vi "收集数据ICRA2024测试椭圆分裂加PID控制.vi"() -> ()   [LabVIEW 2018]
doc: "Demonstrates the use of the Network Streams functions to send LED status to the myRIO target."
uses:
  <vilib>/ErrorRing/Error Ring.xnode
  <vilib>/vision/NI_Vision_Development_Module.lvlib
panel:
  in  "布尔":bool
  in  "ribbon磁场开关":bool=TRUE
  out "控制量":dbl
  in  "期望ratio":dbl=5.0
  in  "拉伸的增益":dbl=10.0
  in  "收缩的增益":dbl=5.0
  in  "predefined control":dbl=5.0
  out "面积":sgl[](array[numeric])
  out "面积":sgl
  out "数据总":dbl[][](array[numeric])
  out "i":i32[](array[numeric])
  out "aspect ratio":dbl[](array[numeric])
  out "D2":i32[](array[numeric])
  out "D1":i32[](array[numeric])
  out "field ratio":sgl[](array[numeric])
  out "field ratio":sgl=4.0
  out "时间":i32
  in  "打开数据记录":bool
  out "aspect ratio":dbl
  out "D2":i32
  out "D1":i32
  out "二值图":T1(plugin-control)
  in  "Search Rect (entire image)":T2={"Left"=200, "Top"=120, "Right"=2000, "Bottom"=1920, "Rotation"=0.0} {"Rotation" format="%.2f"; "Left" scale=0.0..1024.0; "Right" scale=0.0..1024.0}
  out "备用的椭圆角度":sgl
  in  "Number of Erosion":i32=10
  out "Image 7":T1(plugin-control)
  in  "Acquisition Control::Acquisition Frame Rate":dbl=19.50304412841797 min=1.4211589097976685 max=44.94382095336914
  out "Stopped":bool
  in  "Stop (F) 2":bool caption="Stop (F)"
  out "Objects 2":T3(array[cluster]) {"Aspect Ratio" format="%.2f"; "Orientation" format="%.2f"; "Area" format="%.2f"; "Object Center"."Y" format="%.2f"; "Object Center"."X" format="%.2f"}
  in  "Settings 2":T4={"Objects"=0, "Threshold"=128, "Reject Border"=FALSE, "Fill Holes"=FALSE, "Min Object Size"=FALSE, "Min Size"=20000, "Max Object Size"=FALSE, "Max Size"=100, "Show Search Area"=FALSE, "Show Center"=TRUE, "Show Bounding Box"=TRUE} {"Objects" items=["Bright Objects", "Dark Objects"]; "Threshold" min=1 max=999999999 step=1; "Max Size" min=1 max=999999999 step=1; "Min Size" min=1 max=999999999 step=1}
  in  "Range 2":cluster{"Lower value":sgl, "Upper value":sgl}={"Lower value"=0.0, "Upper value"=230.0} {"Upper value" format="%.2f"; "Lower value" format="%.2f"}
  in  "Pause":bool
  out "Array":dbl[](array[numeric])
  in  "Parameter Settings":T5(tab)=enum."Ribbon Oscillating Field" caption="Field Types"
  in  "fg":dbl
  in  "pg":dbl
  in  "dg":dbl
  in  "Ag":dbl
  in  "AoOF":dbl
  in  "fo":sgl
  in  "do":sgl
  in  "oo":sgl
  in  "po":sgl
  in  "cc":sgl
  in  "pc":sgl
  in  "wc":sgl
  in  "dc":sgl
  in  "Ac":dbl
  in  "pr":sgl
  in  "Ar":dbl=8.0
  in  "wr":sgl=18.0
  in  "dr":sgl
  in  "Dis phase step":dbl
  in  "Dis phase frequency (Hz)":dbl
  in  "Dis tumbling frequency (Hz)":dbl
  in  "Dis strength(mT)":dbl
  in  "Swa strength (mT)":dbl
  in  "Swa frequency (Hz)":dbl
  in  "Swa pitch angle (deg)":dbl
  in  "Swa direction angle (deg)":dbl
  in  "Swa ratio":dbl=1.0
  in  "Pitch Angle (rotating around Constant, deg)":dbl
  in  "Ratio (A/C)":sgl=4.0
  in  "Direction Angle (deg)":sgl
  in  "Pitch Angle (rotating around Origin, deg)":sgl
  in  "Frequency (Hz)":sgl=10.0
  in  "Strength (mT)":dbl=10.0
  in  "Ar 2":dbl=5.0 caption="Ar"
  in  "ratio":sgl=1.0
  in  "运动方向":sgl
  in  "长轴方向":sgl
  in  "wr  2":sgl=8.0
  in  "速度大小":sgl
  out "Numeric 5":i32
  in  "Stop":bool
  out "error out":errorcluster
  in  "Target IP Address":string="172.22.11.2"
  # "Overview: Magnetic field calculation, and send parameters to myRIO\nInstructions:\n1. Verify the value of Target IP Address. Set Visa resource name.\n2. Ensure RT Main.vi is already running. \n3. Run this VI. Set parameters of magnetic field."
  # "Strength (mT)"
  # "Pitch Angle (deg)"
  # "Direction Angle (deg)"
  # "Frequency (Hz)"
  # "Strength (mT)"
  # "Oscilation Frequency (Hz)"
  # "Oscilation Angle (deg)"
  # "Pitch Angle (deg)"
  # "Direction Angle (deg)"
  # "Strength (mT)"
  # "Frequency (Hz)"
  # "Pitch Angle (deg)"
  # "Direction Angle (deg)"
  # "Conical Angle (deg)"
  # "Strength (mT)"
  # "Frequency (Hz)"
  # "Pitch Angle (deg)"
  # "Direction Angle (deg)"
  # "Strength (mT)"
  # "Tumbling Frequency (Hz)"
  # "Phase Frequency (Hz)"
  # "Phase Step"
  # "Strength (mT)"
  # "Frequency (Hz)"
  # "Pitch Angle (deg)"
  # "Direction Angle (deg)"
  # "Ratio"
  # "Strength (mT)"
  # "Frequency (Hz)"
  # "Ratio (A/C)"
  # "Direction Angle (deg)"
  # "Pitch Angle (rotating around Origin, deg)"
  # "Pitch Angle (rotating around Constant, deg)"
  # "Strength (mT)"
  # "Frequency (Hz)"
  # "Pitch Angle  (deg)"
  # "longaxis"
  # "Direction Angle (deg)"
  # "ratio (l/s)"
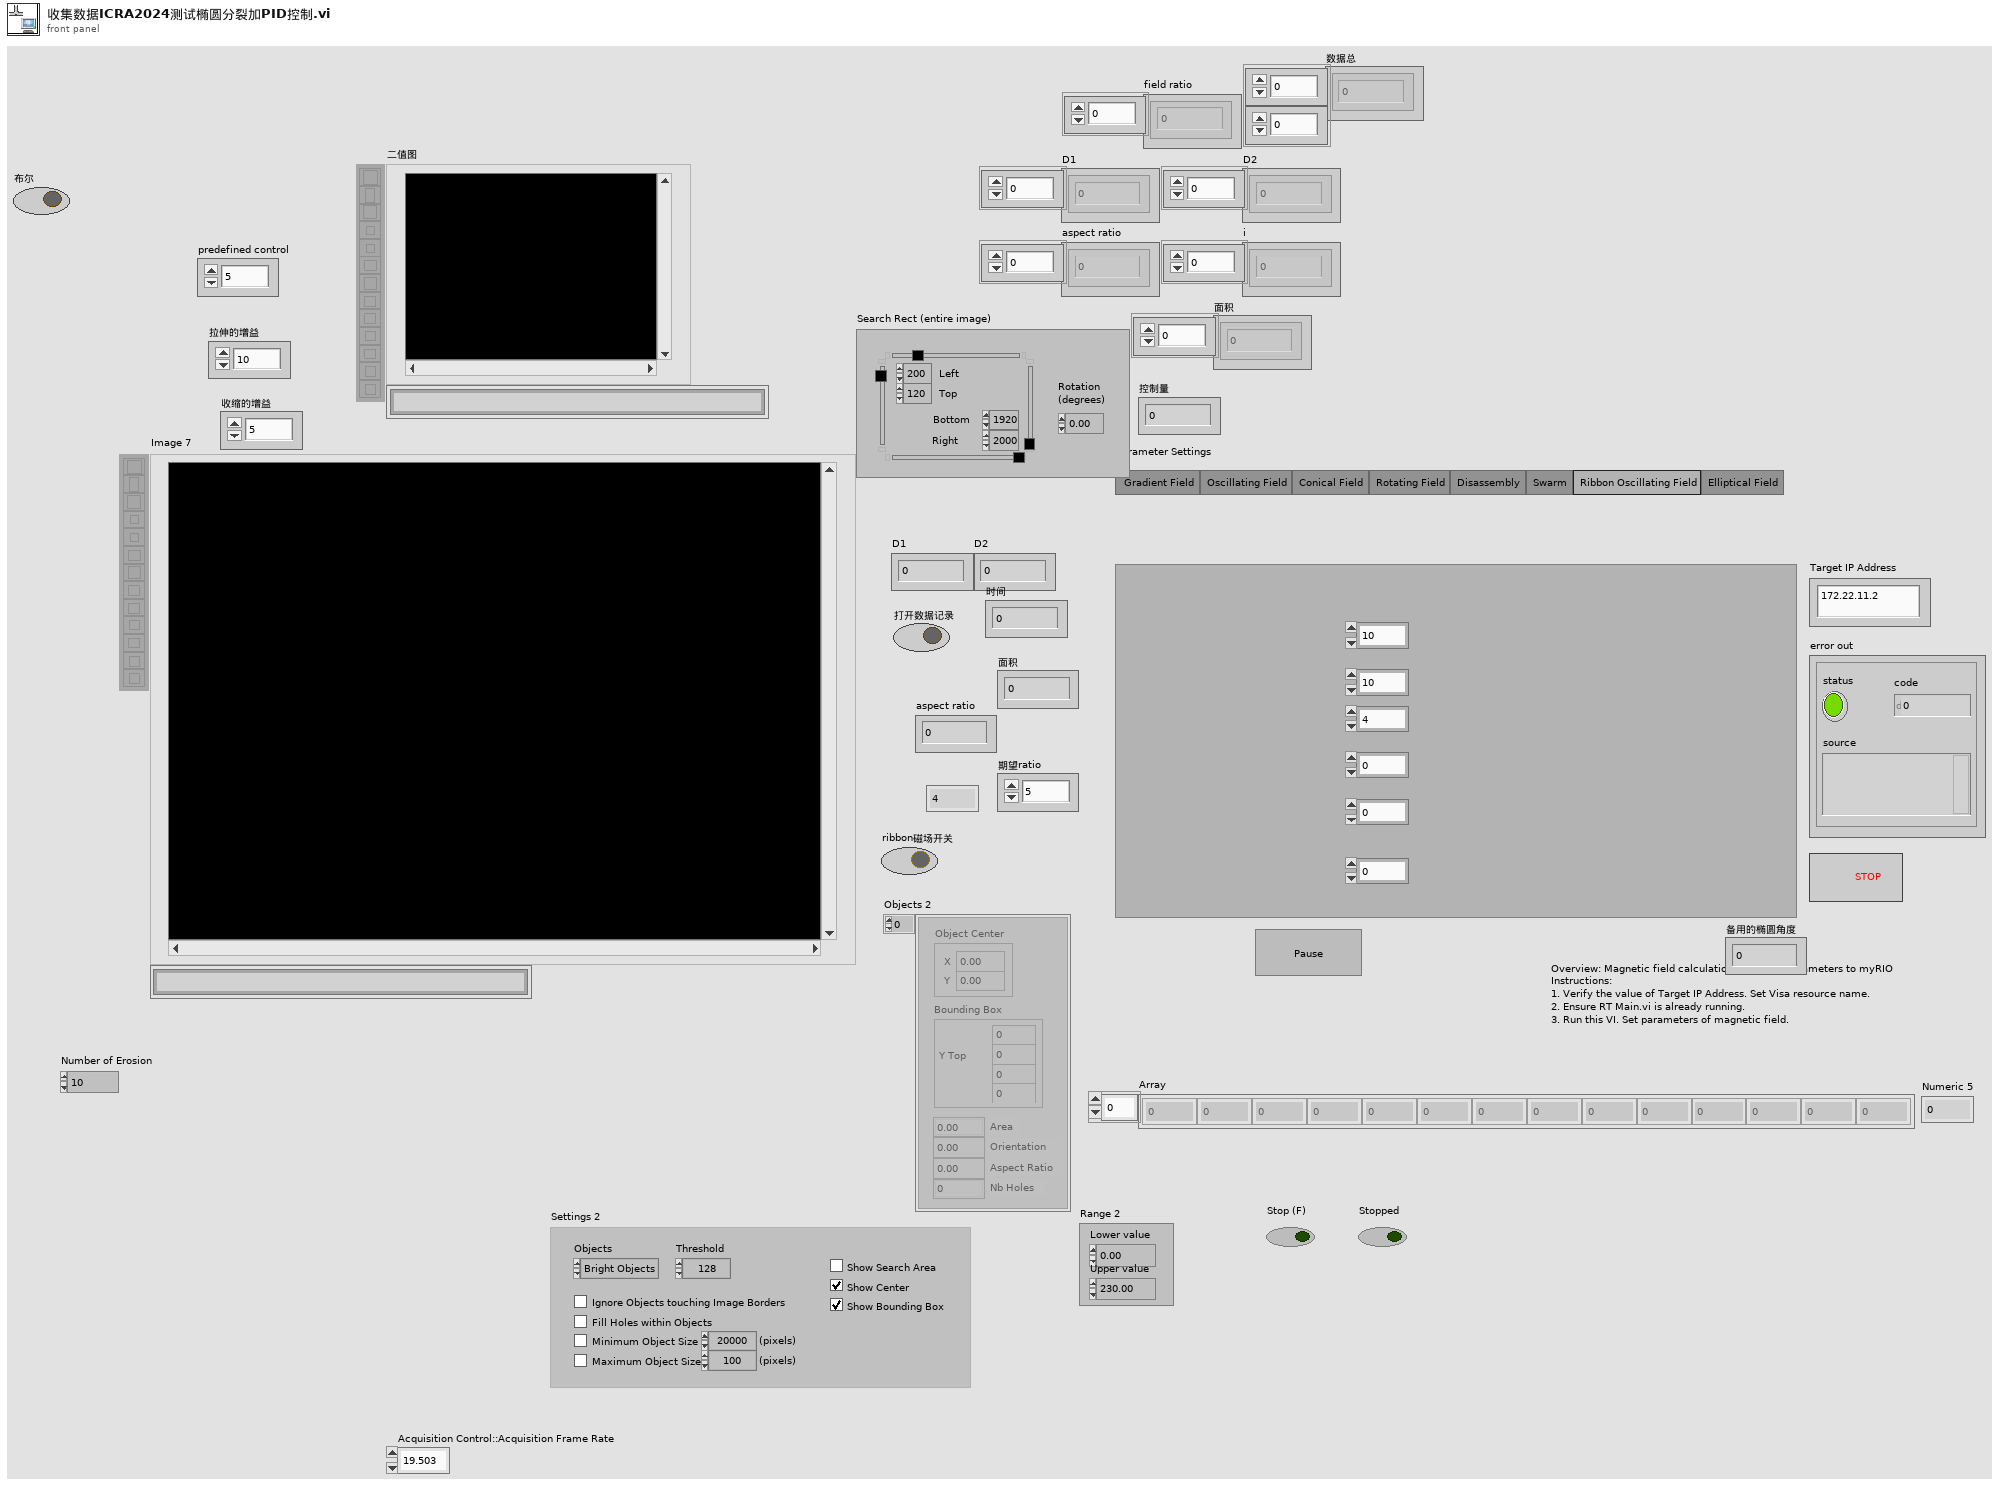
[diagram p1: front panel]
types:
  T1 = typedef "IMAQ Image.ctl" = refnum<image>
  T2 = typedef "IMAQ Rectangle" = cluster{"Left":i32, "Top":i32, "Right":i32, "Bottom":i32, "Rotation":dbl}
  T3 = cluster{"Object Center":cluster{"X":sgl, "Y":sgl}, "Bounding Box":cluster{"X Left":i32, "Y Top":i32, "X Right":i32, "Y Bottom":i32}, "Area":sgl, "Orientation":sgl, "Aspect Ratio":sgl, "Nb Holes":i32}[]
  T4 = cluster{"Objects":u16, "Threshold":i32, "Reject Border":bool, "Fill Holes":bool, "Min Object Size":bool, "Min Size":i32, "Max Object Size":bool, "Max Size":i32, "Show Search Area":bool, "Show Center":bool, "Show Bounding Box":bool}
  T5 = enum32{"Gradient Field ", "Oscillating Field", "Conical Field", "Rotating Field", "Disassembly", "Swarm", "Ribbon Oscillating Field", "Elliptical Field"}
  T6 = typedef "Image Type" = u32
  T7 = cluster{"Objects[0]":cluster{"Object Center":cluster{"X":sgl, "Y":sgl}, "Bounding Box":cluster{"X Left":i32, "Y Top":i32, "X Right":i32, "Y Bottom":i32}, "Area":sgl, "Orientation":sgl, "Aspect Ratio":sgl, "Nb Holes":i32}, "Objects[1]":cluster{"Object Center":cluster{"X":sgl, "Y":sgl}, "Bounding Box":cluster{"X Left":i32, "Y Top":i32, "X Right":i32, "Y Bottom":i32}, "Area":sgl, "Orientation":sgl, "Aspect Ratio":sgl, "Nb Holes":i32}, "Objects[2]":cluster{"Object Center":cluster{"X":sgl, "Y":sgl}, "Bounding Box":cluster{"X Left":i32, "Y Top":i32, "X Right":i32, "Y Bottom":i32}, "Area":sgl, "Orientation":sgl, "Aspect Ratio":sgl, "Nb Holes":i32}, "Objects[3]":cluster{"Object Center":cluster{"X":sgl, "Y":sgl}, "Bounding Box":cluster{"X Left":i32, "Y Top":i32, "X Right":i32, "Y Bottom":i32}, "Area":sgl, "Orientation":sgl, "Aspect Ratio":sgl, "Nb Holes":i32}, "Objects[4]":cluster{"Object Center":cluster{"X":sgl, "Y":sgl}, "Bounding Box":cluster{"X Left":i32, "Y Top":i32, "X Right":i32, "Y Bottom":i32}, "Area":sgl, "Orientation":sgl, "Aspect Ratio":sgl, "Nb Holes":i32}, "Objects[5]":cluster{"Object Center":cluster{"X":sgl, "Y":sgl}, "Bounding Box":cluster{"X Left":i32, "Y Top":i32, "X Right":i32, "Y Bottom":i32}, "Area":sgl, "Orientation":sgl, "Aspect Ratio":sgl, "Nb Holes":i32}, "Objects[6]":cluster{"Object Center":cluster{"X":sgl, "Y":sgl}, "Bounding Box":cluster{"X Left":i32, "Y Top":i32, "X Right":i32, "Y Bottom":i32}, "Area":sgl, "Orientation":sgl, "Aspect Ratio":sgl, "Nb Holes":i32}, "Objects[7]":cluster{"Object Center":cluster{"X":sgl, "Y":sgl}, "Bounding Box":cluster{"X Left":i32, "Y Top":i32, "X Right":i32, "Y Bottom":i32}, "Area":sgl, "Orientation":sgl, "Aspect Ratio":sgl, "Nb Holes":i32}, "Objects[8]":cluster{"Object Center":cluster{"X":sgl, "Y":sgl}, "Bounding Box":cluster{"X Left":i32, "Y Top":i32, "X Right":i32, "Y Bottom":i32}, "Area":sgl, "Orientation":sgl, "Aspect Ratio":sgl, "Nb Holes":i32}}
  T8 = cluster{"Object Center":cluster{"X":sgl, "Y":sgl}, "Bounding Box":cluster{"X Left":i32, "Y Top":i32, "X Right":i32, "Y Bottom":i32}, "Area":sgl, "Orientation":sgl, "Aspect Ratio":sgl, "Nb Holes":i32}
  T9 = cluster{"X Left":i32, "Y Top":i32, "X Right":i32, "Y Bottom":i32}
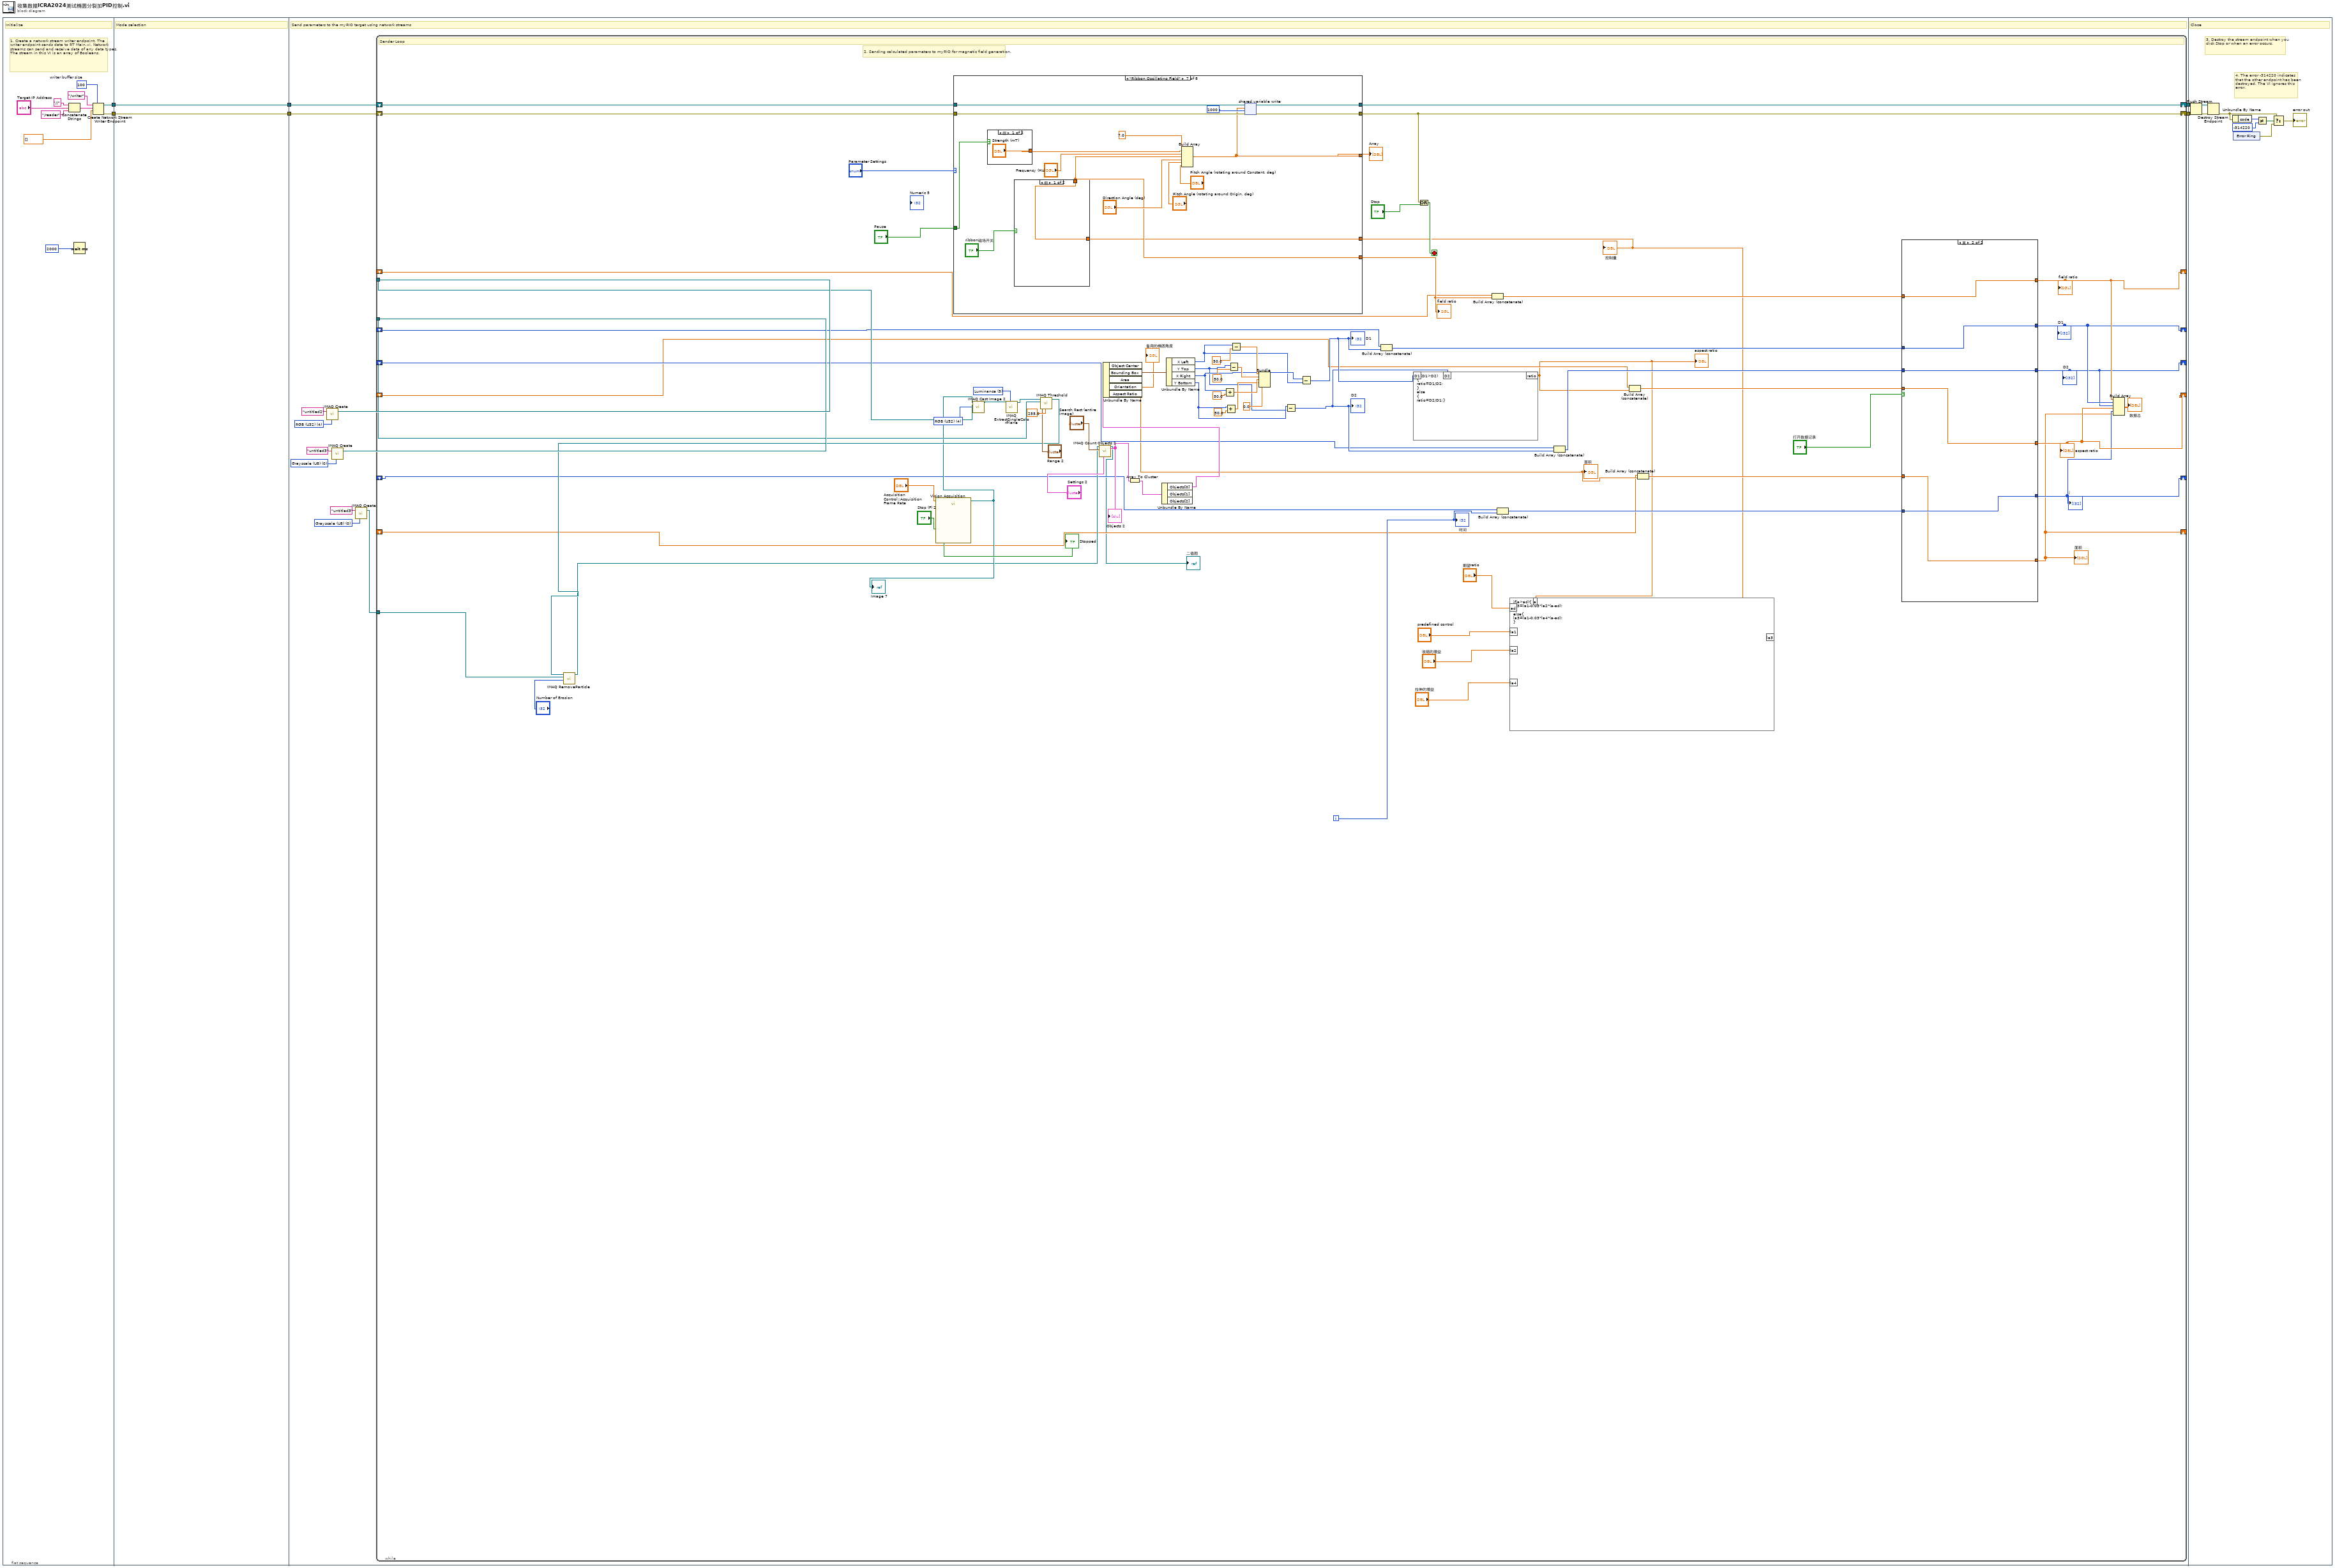
[diagram p0: block diagram]
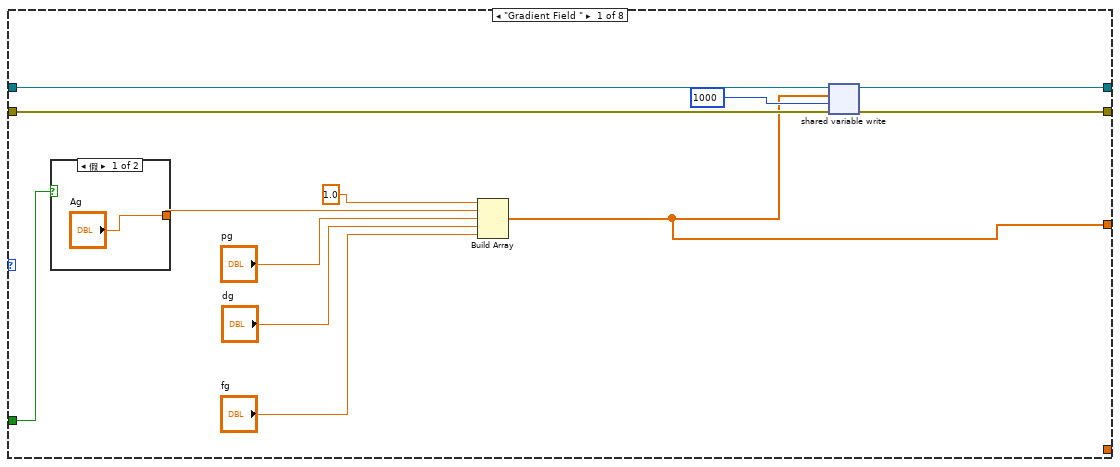
[diagram p3: hidden frame]
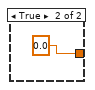
[diagram p4: hidden frame]
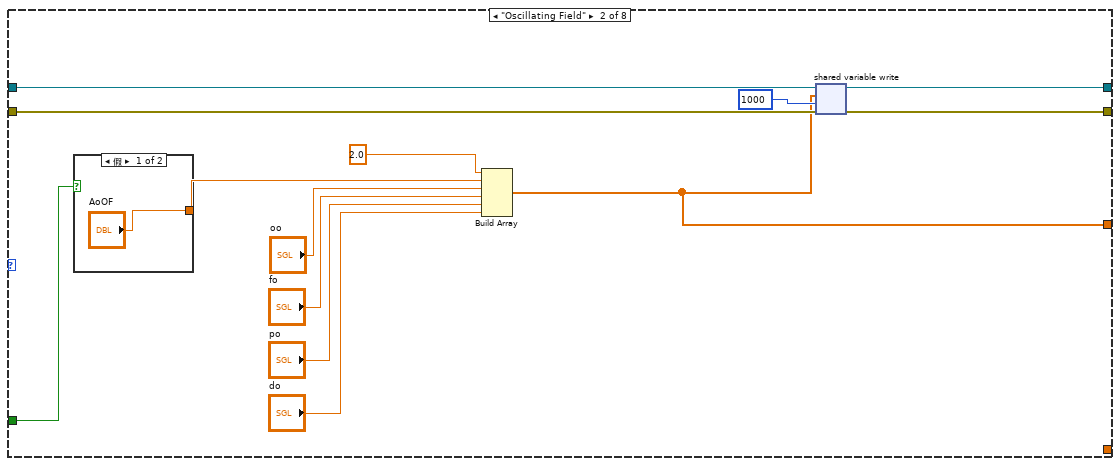
[diagram p5: hidden frame]
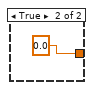
[diagram p6: hidden frame]
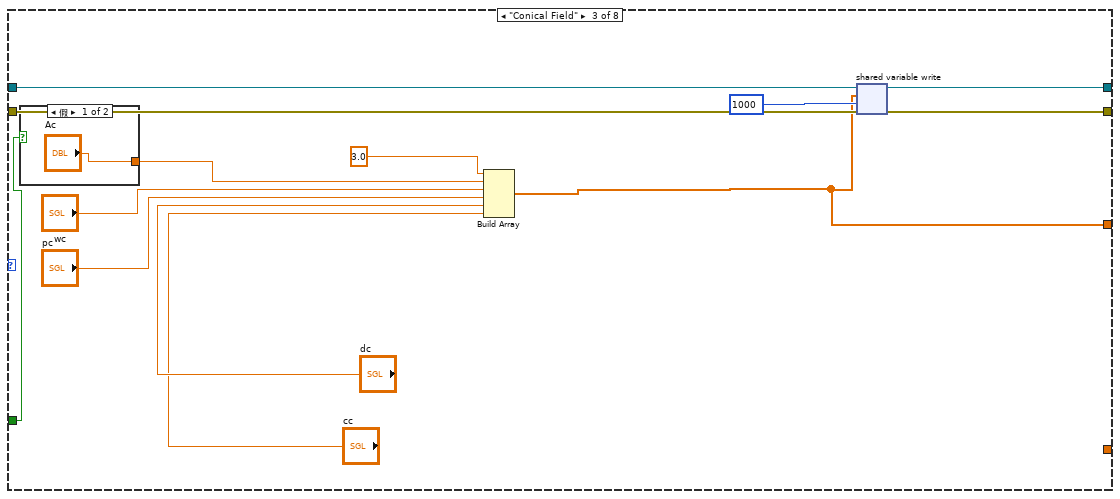
[diagram p7: hidden frame]
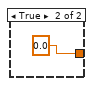
[diagram p8: hidden frame]
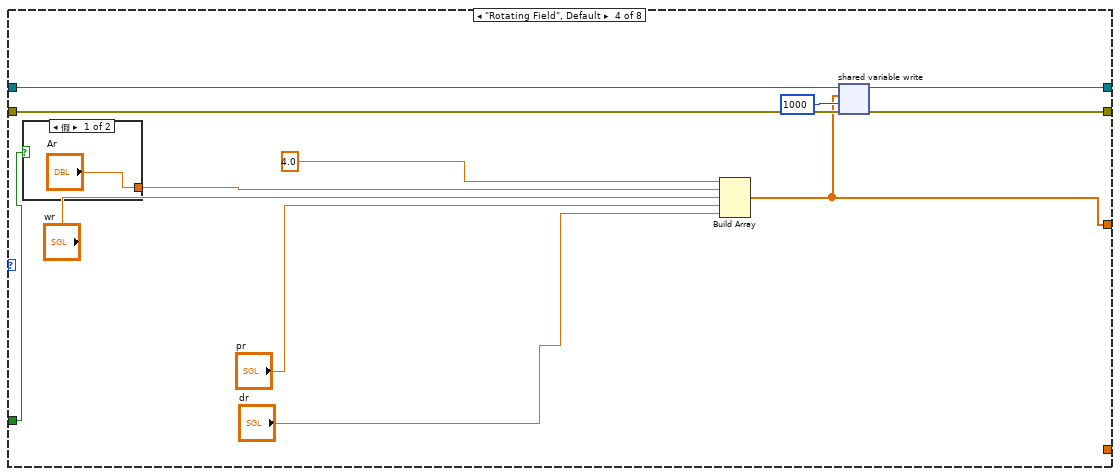
[diagram p9: hidden frame]
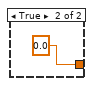
[diagram p10: hidden frame]
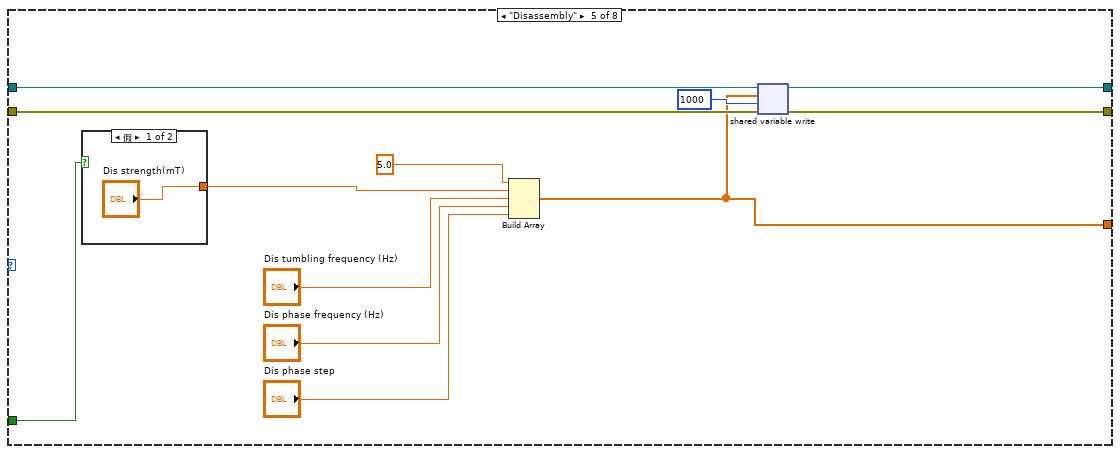
[diagram p11: hidden frame]
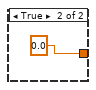
[diagram p12: hidden frame]
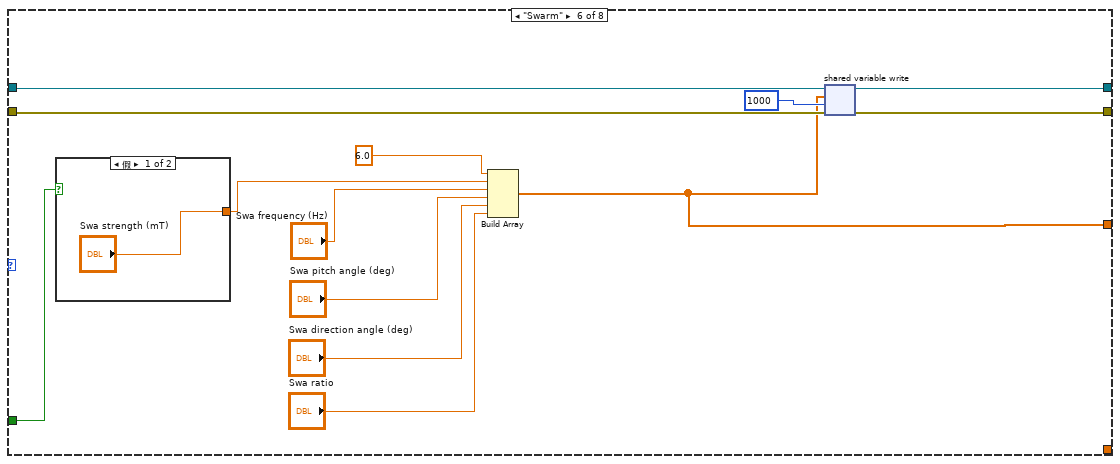
[diagram p13: hidden frame]
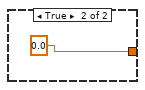
[diagram p14: hidden frame]
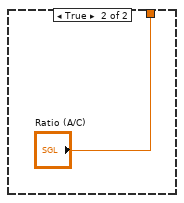
[diagram p15: hidden frame]
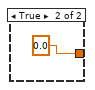
[diagram p16: hidden frame]
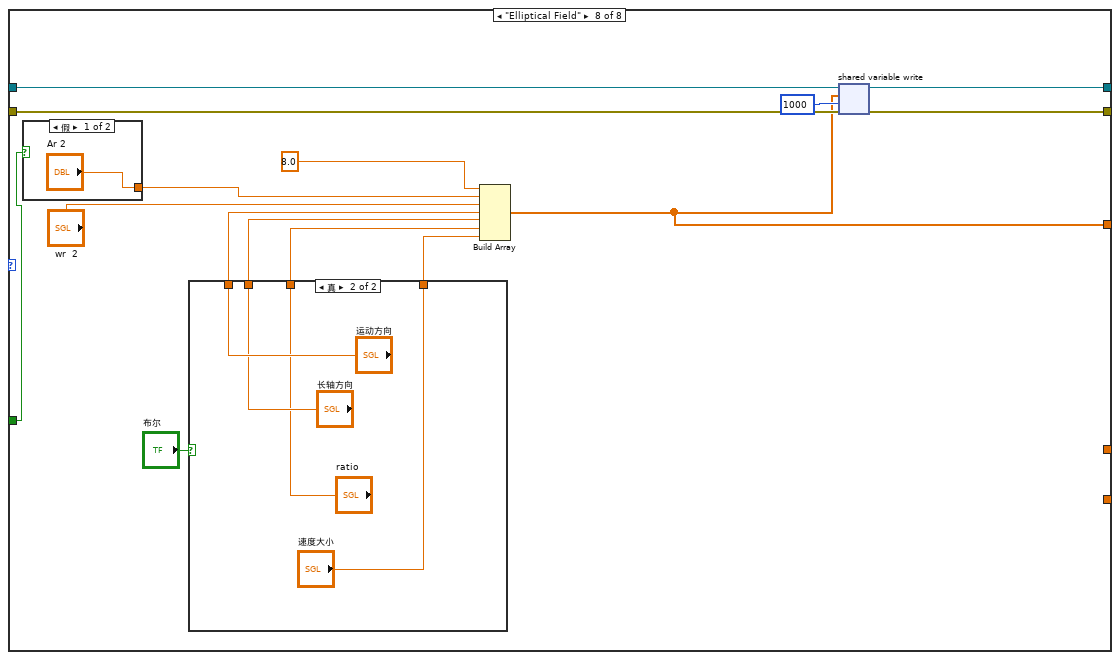
[diagram p17: hidden frame]
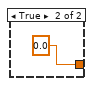
[diagram p19: hidden frame]
diagram:
  n1 = flat-sequence {
    tunnel: [w11] -> w2
    tunnel: [w10] -> w1
    tunnel: [w18] -> w4
    tunnel: [w17] -> w3
    tunnel: w1 -> [w17]
    tunnel: w2 -> [w18]
    tunnel: [w29] -> w6
    tunnel: w4 -> [w31]
    tunnel: [w28] -> w5
    tunnel: w3 -> [w30]
    tunnel: w6 -> [w252]
    tunnel: w5 -> [w249]
    frame #0 {
      w9 = 100  # writer buffer size
      # "1. Create a network stream writer endpoint. The writer endpoint sends data to RT Main.vi. Network streams can send and receive data of any data types. The stream in this VI is an array of Booleans."
      # "Initialize"
      n2 = Concatenate Strings("//", "Target IP Address", "/reader") -> (w16:string)
      n3 = Wait (ms)(milliseconds to wait=2000) -> ()  [unwired: 1 out]
      n4 = Create Network Stream Writer Endpoint(7:w9, 9:dbl[] [], 10:w16, 11:"/writer" ("reader name")) -> (0:w10:errorcluster, 3:w11:refnum<k21>)  [unwired: 3 in]
    }
    frame #1 {
      # "Mode selection"
    }
    frame #2 {
      w20 = T6 0 items=["Grayscale (U8)", "Grayscale (I16)", "Grayscale (SGL)", "Complex (CSG)", "RGB (U32)", "HSL (U32)", "RGB (U64)", "Grayscale (U16)"] ("Image Type")
      w24 = T6 0 items=["Grayscale (U8)", "Grayscale (I16)", "Grayscale (SGL)", "Complex (CSG)", "RGB (U32)", "HSL (U32)", "RGB (U64)", "Grayscale (U16)"] ("Image Type")
      w26 = T6 4 items=["Grayscale (U8)", "Grayscale (I16)", "Grayscale (SGL)", "Complex (CSG)", "RGB (U32)", "HSL (U32)", "RGB (U64)", "Grayscale (U16)"] ("Image Type")
      # "Send parameters to the myRIO target using network streams"
      n5 = call "IMAQ Create"("Image Name"="untitled2", "Image Type"=w26) -> ("New Image"=w23:T1)  [unwired: 3 in, 1 out]
      n6 = call "IMAQ Create"("Image Name"="untitled3", "Image Type"=w24) -> ("New Image"=w22:T1)  [unwired: 3 in, 1 out]
      n7 = call "IMAQ Create"("Image Name"="untitled3", "Image Type"=w20) -> ("New Image"=w19:T1)  [unwired: 3 in, 1 out]
      n8 = while {
        shift-right: [w104] -> w28
        shift-left: w30 -> [w106]
        shift-right: [w105] -> w29
        shift-left: w31 -> [w107]
        tunnel: w22 -> [w95]
        tunnel: w23 -> [w90]
        tunnel: w19 -> [w75]
        shift-right: [w48] -> _
        shift-left: _ -> [w60]
        shift-right: [w47] -> _
        shift-left: _ -> [w57]
        shift-right: [w46] -> _
        shift-left: _ -> [w54]
        shift-right: [w45] -> _
        shift-left: _ -> [w52]
        shift-right: [w44] -> _
        shift-left: _ -> [w49]
        shift-right: [w40] -> _
        shift-left: _ -> [w39]
        i -> [w51]
        stop <- w94 stop-if-true
        w89 = T6 4 items=["Grayscale (U8)", "Grayscale (I16)", "Grayscale (SGL)", "Complex (CSG)", "RGB (U32)", "HSL (U32)", "RGB (U64)", "Grayscale (U16)"] ("Image Type")
        w100 = 5 items=["Red", "Green", "Blue", "Hue", "Saturation", "Luminance", "Value", "Intensity"] ("Color Plane")
        # "2. Sending calculated parameters to myRIO for magnetic field generation."
        # "Sender Loop"
        n9 = call "Vision Acquisition"("Acquisition Control::Acquisition Frame Rate"="Acquisition Control::Acquisition Frame Rate", "Stop (F)"="Stop (F) 2") -> ("Image Out"=w67:T1, "Stopped"=→"Stopped":bool)  [unwired: 23 in, 1 out]
        "Image 7" <- w67
        n10 = call "IMAQ Cast Image 2"("Image Src"=w67, "Image Dst"=w90, "Image Type"=w89) -> ("Image Dst Out"=w91:T1)  [unwired: 11 in, 1 out]
        n11 = call "IMAQ ExtractSingleColorPlane"("Color Plane"=w100, "Image Src"=w91) -> ("Image Dst Out"=w73:T1)  [unwired: 8 in, 1 out]
        n12 = call "IMAQ Threshold"("Replace Value"=sgl 255.0, "Range"="Range 2", "Image Dst"=w95, "Image Src"=w73) -> ("Image Dst Out"=w76:T1)  [unwired: 6 in, 1 out]
        n13 = call "IMAQ RemoveParticle"("Number of Erosion"="Number of Erosion", "Image Dst"=w75, "Image Src"=w76) -> ("Image Dst Out"=w66:T1)  [unwired: 7 in, 1 out]
        n14 = call "IMAQ Count Objects 2"("Settings"="Settings 2", "Search Rect (entire image)"="Search Rect (entire image)", "Image"=w66) -> ("Image Out"=→"二值图":T1, "Objects"=w96:T3)  [unwired: 4 in, 3 out]
        "Objects 2" <- w96
        n15 = Array To Cluster(array=w96) -> (cluster=w78:T7)
        n16 = Unbundle By Name(w78) -> ("Objects[0]"=w77:T8)  [unwired: 2 out]
        n17 = Unbundle By Name(w77) -> ("Bounding Box"=w88:T9, "Area"=w42:sgl, "Orientation"=→"备用的椭圆角度":sgl)  [unwired: 2 out]
        "面积" <- w42
        n18 = Unbundle By Name(w88) -> ("X Left"=w69:i32, "Y Top"=w64:i32, "X Right"=w70:i32, "Y Bottom"=w65:i32)
        n19 = Add(x=w70, y=50.0) -> (x+y=w81:dbl)
        n20 = Add(x=w65, y=50.0) -> (x+y=w80:dbl)
        n21 = Subtract(x=w64, y=50.0) -> (x-y=w82:dbl)
        n22 = Subtract(x=w69, y=50.0) -> (x-y=w83:dbl)
        n23 = Bundle(w83, w82, w81, w80, 0.0) -> ()  [unwired: 1 in, 1 out]
        n24 = Subtract(x=w65, y=w64) -> (x-y=w56:i32)
        "D2" <- w56
        n25 = Subtract(x=w70, y=w69) -> (x-y=w59:i32)
        "D1" <- w59
        n26 = Build Array (concatenate)(w57, w59) -> (w58:i32[])
        n27 = formula code="if (D1>D2)\n{\nratio=D1/D2;\n}\nelse\n{\nratio=D2/D1;}"("D1"=w59, "D2"=w56) -> ("ratio"=w34:dbl)
        "aspect ratio" <- w34
        n28 = Build Array (concatenate)(w49, w51) -> (w50:i32[])
        n29 = formula code="if(a>ad){\nla3=la1-0.03*la2*(a-ad);\n}\nelse{\nla3=la1-0.03*la4*(a-ad);\n}"("ad"="期望ratio", "a"=w34, "la1"="predefined control", "la2"="收缩的增益", "la4"="拉伸的增益") -> ("la3"=w32:dbl)
        "控制量" <- w32
        n30 = case shown="\"Ribbon Oscillating Field\"" "Parameter Settings" {
          tunnel: w107 -> [w125 w140 w155 w169 w183 w197 w217 w235]
          tunnel: w106 -> [w122 w139 w154 w168 w181 w196 w215 w234]
          tunnel: [w124 w138 w152 w167 w182 w195 w216 w233] -> w105
          tunnel: [w123 w137 w153 w166 w180 w194 w214 w232] -> w104
          tunnel: [w118 w131 w146 w161 w174 w189 w212 w227] -> w103
          tunnel: "Pause" -> [w116 w129 w144 w159 w173 w188 w208 w225]
          tunnel: [_ _ _ _ _ _ w205 _] -> w62
          tunnel: w32 -> [_ _ _ _ _ _ w203 _]
          frame "Gradient Field " {
            n31 = case shown="假" w116 {
              tunnel: ["Ag" 0.0] -> w117
              frame False {
              }
              frame True {
              }
            }
            n32 = Build Array(1.0, w117, "pg", "dg", "fg") -> (w118:dbl[])
            n33 = shared-variable-write(w125, w122, w118, 1000 ("timeout ms (-1)")) -> (w124:refnum<k21>, w123:errorcluster)  [unwired: 1 out]
          }
          frame "Oscillating Field" {
            n34 = case shown="假" w129 {
              tunnel: ["AoOF" 0.0] -> w130
              frame False {
              }
              frame True {
              }
            }
            n35 = Build Array(2.0, w130, "oo", "fo", "po", "do") -> (w131:dbl[])
            n36 = shared-variable-write(w140, w139, w131, 1000 ("timeout ms (-1)")) -> (w138:refnum<k21>, w137:errorcluster)  [unwired: 1 out]
          }
          frame "Conical Field" {
            # "FG"
            n37 = case shown="假" w144 {
              tunnel: ["Ac" 0.0] -> w145
              frame False {
              }
              frame True {
              }
            }
            n38 = Build Array(3.0, w145, "wc", "pc", "dc", "cc") -> (w146:dbl[])
            n39 = shared-variable-write(w155, w154, w146, 1000 ("timeout ms (-1)")) -> (w152:refnum<k21>, w153:errorcluster)  [unwired: 1 out]
          }
          frame "Rotating Field", Default {
            n40 = case shown="假" w159 {
              tunnel: ["Ar" 0.0] -> w160
              frame False {
              }
              frame True {
              }
            }
            n41 = Build Array(4.0, w160, "wr", "pr", "dr") -> (w161:dbl[])
            n42 = shared-variable-write(w169, w168, w161, 1000 ("timeout ms (-1)")) -> (w167:refnum<k21>, w166:errorcluster)  [unwired: 1 out]
          }
          frame "Disassembly" {
            n43 = case shown="假" w173 {
              tunnel: ["Dis strength(mT)" 0.0] -> w178
              frame False {
              }
              frame True {
              }
            }
            n44 = Build Array(5.0, w178, "Dis tumbling frequency (Hz)", "Dis phase frequency (Hz)", "Dis phase step") -> (w174:dbl[])
            n45 = shared-variable-write(w183, w181, w174, 1000 ("timeout ms (-1)")) -> (w182:refnum<k21>, w180:errorcluster)  [unwired: 1 out]
          }
          frame "Swarm" {
            n46 = case shown="假" w188 {
              tunnel: ["Swa strength (mT)" 0.0] -> w187
              frame False {
              }
              frame True {
              }
            }
            n47 = Build Array(6.0, w187, "Swa frequency (Hz)", "Swa pitch angle (deg)", "Swa direction angle (deg)", "Swa ratio") -> (w189:dbl[])
            n48 = shared-variable-write(w197, w196, w189, 1000 ("timeout ms (-1)")) -> (w195:refnum<k21>, w194:errorcluster)  [unwired: 1 out]
          }
          frame "Ribbon Oscillating Field" {
            n49 = case shown="假" w208 {
              tunnel: ["Strength (mT)" 0.0] -> w207
              frame False {
              }
              frame True {
              }
            }
            n50 = case shown="假" "ribbon磁场开关" {
              tunnel: [w218 "Ratio (A/C)"] -> w205
              tunnel: w203 -> [w218 _]
              frame False {
              }
              frame True {
              }
            }
            n51 = Build Array(7.0, w207, "Frequency (Hz)", w205, "Direction Angle (deg)", "Pitch Angle (rotating around Origin, deg)", "Pitch Angle (rotating around Constant, deg)") -> (w212:dbl[])
            n52 = shared-variable-write(w217, w215, w212, 1000 ("timeout ms (-1)")) -> (w216:refnum<k21>, w214:errorcluster)  [unwired: 1 out]
          }
          frame "Elliptical Field" {
            n53 = case shown="假" w225 {
              tunnel: ["Ar 2" 0.0] -> w226
              frame False {
              }
              frame True {
              }
            }
            n54 = case shown="真" "布尔" {
              tunnel: [_ "运动方向"] -> w230
              tunnel: [_ "长轴方向"] -> w229
              tunnel: [_ "ratio"] -> w224
              tunnel: [_ "速度大小"] -> w223
              frame False {
              }
              frame True {
              }
            }
            n55 = Build Array(8.0, w226, "wr  2", w230, w229, w224, w223) -> (w227:dbl[])
            n56 = shared-variable-write(w235, w234, w227, 1000 ("timeout ms (-1)")) -> (w233:refnum<k21>, w232:errorcluster)  [unwired: 1 out]
          }
        }
        "Array" <- w103
        "field ratio" <- w62
        n57 = Or(x=w104, y="Stop") -> (x .or. y?=w94:bool)
        n58 = Build Array (concatenate)(w60, w62) -> (w61:dbl[])
        n59 = Build Array (concatenate)(w54, w56) -> (w55:i32[])
        n60 = Build Array (concatenate)(w52, w34) -> (w53:dbl[])
        n61 = Build Array (concatenate)(w39, w42) -> (w41:sgl[])
        n62 = case shown="真" "打开数据记录" {
          tunnel: [_ w114] -> w48
          tunnel: w61 -> [_ w114]
          tunnel: [_ w113] -> w47
          tunnel: w58 -> [_ w113]
          tunnel: [_ w112] -> w46
          tunnel: w55 -> [_ w112]
          tunnel: [_ w111] -> w45
          tunnel: w53 -> [_ w111]
          tunnel: [_ w110] -> w44
          tunnel: w50 -> [_ w110]
          tunnel: [_ w109] -> w40
          tunnel: w41 -> [_ w109]
          frame False {
          }
          frame True {
          }
        }
        "field ratio" <- w48
        "D1" <- w47
        "D2" <- w46
        "aspect ratio" <- w45
        "i" <- w44
        "面积" <- w40
        n63 = Build Array(w48, w47, w46, w45, w44, w40) -> (→"数据总":dbl[][])
        "时间" <- w51
      }
    }
    frame #3 {
      # "4. The error -314220 indicates that the other endpoint has been destroyed. The VI ignores this error."
      # "3. Destroy the stream endpoint when you click Stop or when an error occurs."
      # "Close"
      n64 = Flush Stream(8:w249, 11:w252) -> (0:w250:errorcluster, 3:w251:refnum<k21>)  [unwired: 2 in, 1 out]
      n65 = Destroy Stream Endpoint(8:w250, 11:w251) -> (0:w244:errorcluster)
      n66 = Unbundle By Name(w244) -> ("code"=w248:i32)
      n67 = xnode "Error Ring"() -> ("错误输出"=w245:errorcluster)
      n68 = Not Equal?(x=w248, y=-314220) -> (x != y?=w246:bool)
      n69 = Select(t=w244, s=w246, f=w245) -> (s? t:f=→"error out":errorcluster)
    }
  }
